vi "ParseVariantCovers.vi"(9 "Covers Not Found?":bool, 10 "CoversSubSection":string) -> (3 "VariantCovers":T1[](array[typedef]))   [LabVIEW 2022 SP3]
uses:
  TypeDefs/Variant.ctl
  <vilib>/Utility/error.llb/Trim Whitespace One-Sided.vi
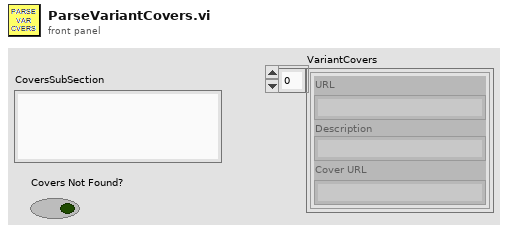
[diagram p1: front panel]
types:
  T1 = typedef "Variant.ctl" = cluster{"URL":string, "Description":string, "Cover URL":string}
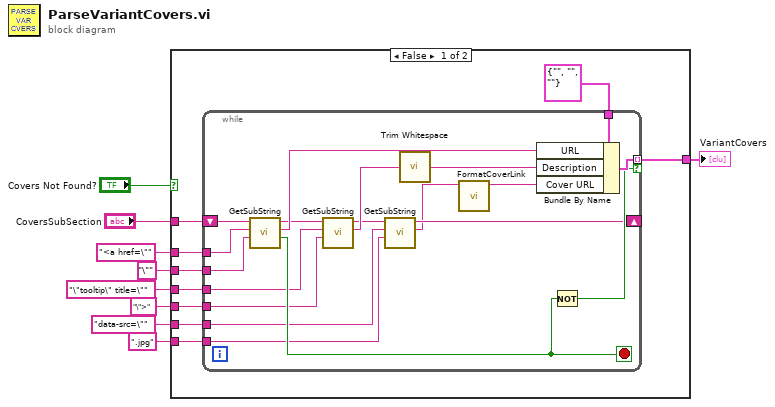
[diagram p0: block diagram]
diagram:
  n1 = case shown="False" "Covers Not Found?" {
    tunnel: "CoversSubSection" -> [w18 _]
    tunnel: "<a href=\"" -> [w17 _]
    tunnel: "\"" -> [w16 _]
    tunnel: [w14 _] -> w5
    tunnel: "\"tooltip\" title=\"" -> [w13 _]
    tunnel: "\">" -> [w12 _]
    tunnel: "data-src=\"" -> [w11 _]
    tunnel: ".jpg" -> [w10 _]
    frame False {
      n2 = while {
        shift-right: [w21] -> _
        shift-left: w18 -> [w37]
        tunnel: w17 -> [w36]
        tunnel: w16 -> [w35]
        tunnel: T1 {"URL"="", "Description"="", "Cover URL"=""} ("Variant Covers") -> [w34]
        tunnel: [w33] -> w14 mode=indexing if=w31
        tunnel: w13 -> [w28]
        tunnel: w12 -> [w27]
        tunnel: w11 -> [w23]
        tunnel: w10 -> [w22]
        stop <- w32 stop-if-true
        n3 = call "GetSubString.vi"("End Search"=w35, "Start Search"=w36, "String In"=w37) -> ("Not Found?"=w32:bool, "Match"=w30:string, "Following String Out"=w29:string)  [unwired: 6 in]
        n4 = call "GetSubString.vi"("End Search"=w27, "Start Search"=w28, "String In"=w29) -> ("Match"=w26:string, "Following String Out"=w24:string)  [unwired: 6 in, 1 out]
        n5 = call "GetSubString.vi"("End Search"=w22, "Start Search"=w23, "String In"=w24) -> ("Match"=w20:string, "Following String Out"=w21:string)  [unwired: 6 in, 1 out]
        n6 = call <vilib>:"Trim Whitespace.vi"("string"=w26) -> ("trimmed string"=w25:string)  [unwired: 1 in]
        n7 = call "FormatCoverLink.vi"("Cover Link"=w20) -> ("result string"=w19:string)  [unwired: 10 in]
        n8 = Bundle By Name(cluster=w34, "URL"=w30, "Description"=w25, "Cover URL"=w19) -> (w33:T1)
        n9 = Not(x=w32) -> (.not. x?=w31:bool)
      }
    }
    frame True {
    }
  }
  "VariantCovers" <- w5
